vi "Calc - ThetaB.vi"(11 "TBMeas":dbl) -> (3 "ThetaB":dbl)   [LabVIEW 2018, in "Controller (Host).lvlib"]
uses:
  Controller (Host).lvlib
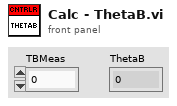
[diagram p1: front panel]
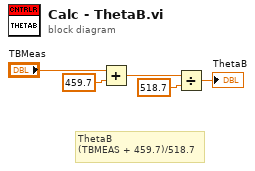
[diagram p0: block diagram]
diagram:
  # "ThetaB\n(TBMEAS + 459.7)/518.7"
  n1 = Add(x="TBMeas", y=459.7) -> (x+y=w2:dbl)
  n2 = Divide(x=w2, y=518.7) -> (x/y=→"ThetaB":dbl)
